vi "Read Model constants.vi"(11 "CurrentToField in":refnum<class "CurrentToField.lvclass">) -> (2 "Model constants":T1, 3 "CurrentToField out":refnum<class "CurrentToField.lvclass">)   [LabVIEW 2020, in "CurrentToField.lvclass"]
uses:
  CurrentToField.lvclass
  CurrentToField.lvclass/CurrentToField.ctl
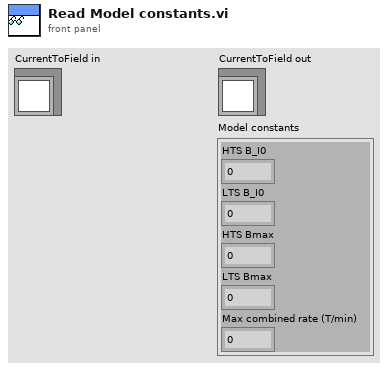
[diagram p1: front panel]
types:
  T1 = cluster{"HTS B_I0":dbl, "LTS B_I0":dbl, "HTS Bmax":dbl, "LTS Bmax":dbl, "Max combined rate (T/min)":dbl}
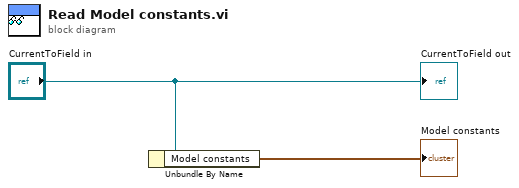
[diagram p0: block diagram]
diagram:
  n1 = Unbundle By Name("CurrentToField in") -> ("Model constants"=→"Model constants":T1)
  "CurrentToField out" <- "CurrentToField in"
